vi "Main.vi"(8 "error in (no error)":errorcluster, 11 "Retiga in":refnum<class "Retiga.lvclass">) -> (0 "error out":errorcluster, 3 "component":refnum<class "Retiga.lvclass">)   [LabVIEW 2012, in "Retiga.lvclass"]
doc: "Main VI of the component. This should contain the GUI of your component and be called when creating an executable."
uses:
  Retiga.lvclass
  <vilib>/Distrio/Murmex/Murmex/command_enum.ctl
  <vilib>/Distrio/Murmex/InitialiseMessage/InitialiseMessage.lvclass
  <vilib>/Distrio/Murmex/TerminateMessage/TerminateMessage.lvclass
  <vilib>/Distrio/Murmex/ConfigureMessage/ConfigureMessage.lvclass
  <vilib>/Distrio/Murmex/StopMessage/StopMessage.lvclass
  <vilib>/Distrio/Murmex/StartMessage/StartMessage.lvclass
  <vilib>/Distrio/Murmex/Murmex/update_cluster.ctl
  <vilib>/Distrio/Murmex/GenericMessage/GenericMessage.lvclass
  Retiga.lvclass/Retiga.ctl
  <vilib>/Distrio/Murmex/Murmex/Murmex.lvclass
  <vilib>/Distrio/Murmex/Murmex/Set configure at initialise.vi
  <vilib>/Distrio/Murmex/Murmex/Set log reference.vi
  <vilib>/Distrio/Murmex/Murmex/Set VI reference.vi
  <vilib>/Distrio/Murmex/Murmex/Get ID.vi
  <vilib>/Distrio/Murmex/Murmex/Set write log to disk.vi
  <vilib>/Distrio/Murmex/Message/Add or replace parameter.vi
  <vilib>/Distrio/Murmex/Message/Message.lvclass
panel:
  in  "PID gains":T1
  out "terminate?":bool
  in  "button:configure":bool
  in  "button:quit":bool
  in  "Tab Control":enum32{"Focus", "Phase comparison", "Debug"}(tab)
  in  "button:select_rois":bool
  in  "button:save":bool
  in  "button:start":bool
  in  "File Name":string
  in  "Base Path":path
  in  "Exposure (us)":i32
  in  "Gain":i32
  out "Focus":T2(plugin-control)
  out "av. translation":dbl[unit]
  in  "button:send move":bool
  in  "button:autofocus":bool
  in  "button:set as focus":bool
  out "aligned":T2(plugin-control)
  out "roy":T2(plugin-control)
  out "rob":T2(plugin-control)
  out "ROY":T2(plugin-control)
  out "ROB":T2(plugin-control)
  out "good alignment?":bool
  out "translation":dbl[unit]
  out "pixel shift":dbl
  out "log":string
  in  "Component id":string="Retiga"
  in  "command":T3
  in  "generic command":string
  in  "button:send command":bool
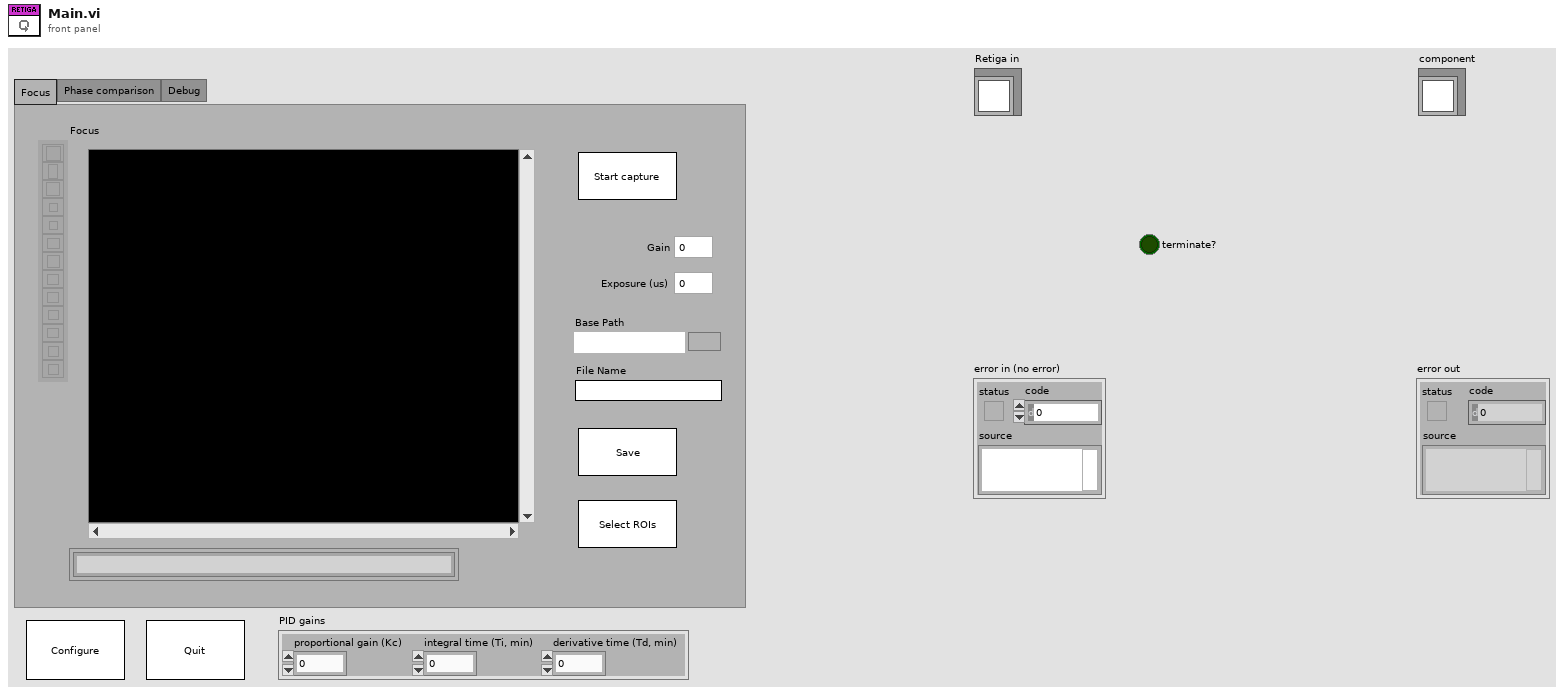
[diagram p1: front panel]
types:
  T1 = cluster{"proportional gain (Kc)":dbl, "integral time (Ti, min)":dbl, "derivative time (Td, min)":dbl}
  T2 = typedef "IMAQ Image.ctl" = refnum<image>
  T3 = typedef "Murmex.lvlib/Murmex.lvclass/command_enum.ctl" = enum16{"null", "initialise", "reset", "terminate", "acknowledge", "update", "inspect", "inform", "proceed", "start", "stop", "fetch", "configure", "generic"}
  T4 = enum8{"Enabled", "Disabled", "Disabled and Grayed Out"}
  T5 = typedef "Murmex.lvlib/Murmex.lvclass/update_cluster.ctl" = cluster{"target ID":string, "key chains":string[], "values":variant[]}
  T6 = typedef "Murmex.lvclass/command_enum.ctl" = enum16{"null", "initialise", "reset", "terminate", "acknowledge", "update", "inspect", "inform", "proceed", "start", "stop", "fetch", "configure", "generic"}
  T7 = typedef "Murmex.lvclass/Event type enumerations.ctl" = enum16{"before", "after"}
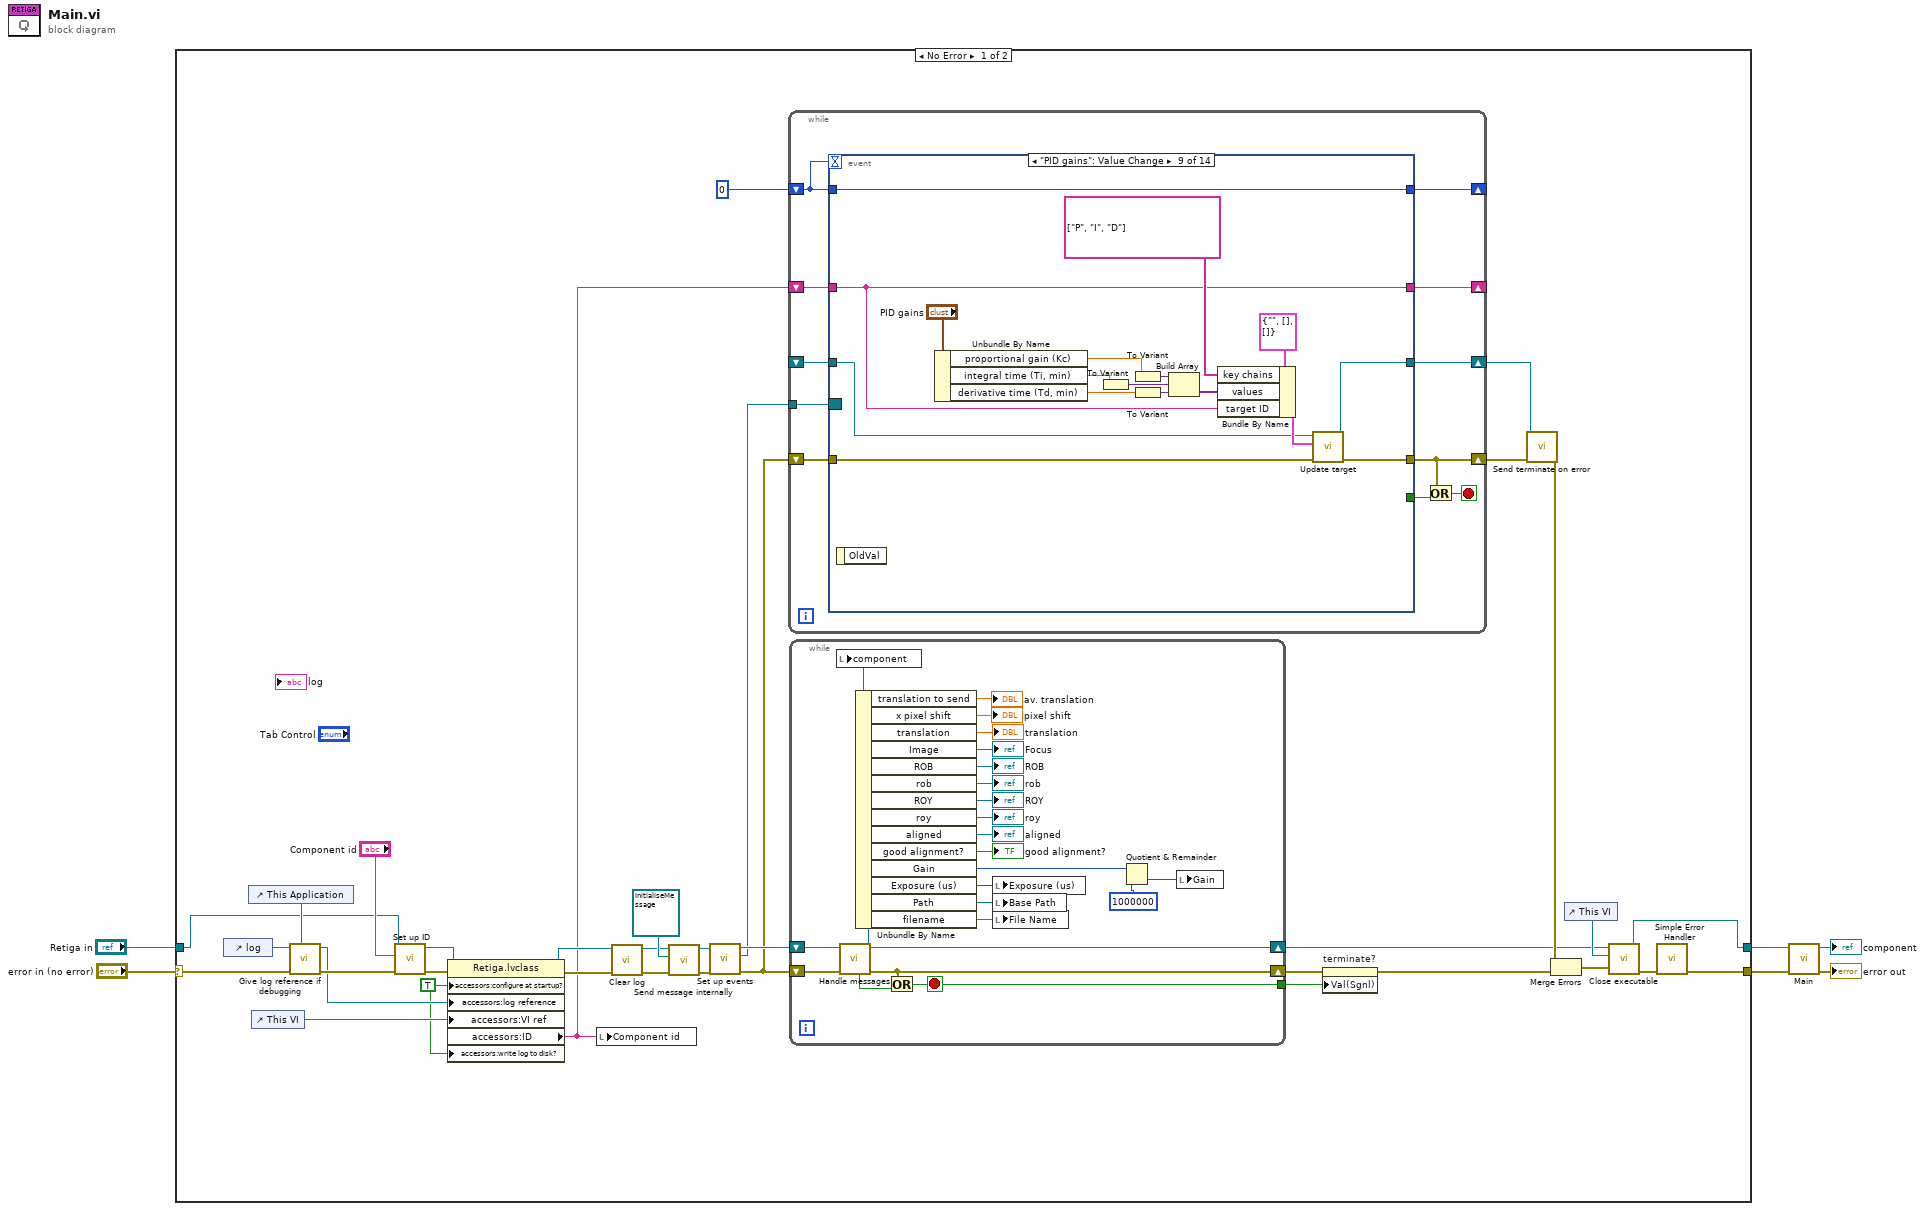
[diagram p0: block diagram]
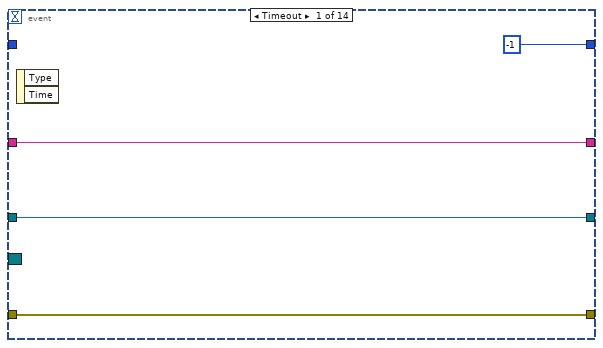
[diagram p2: hidden frame]
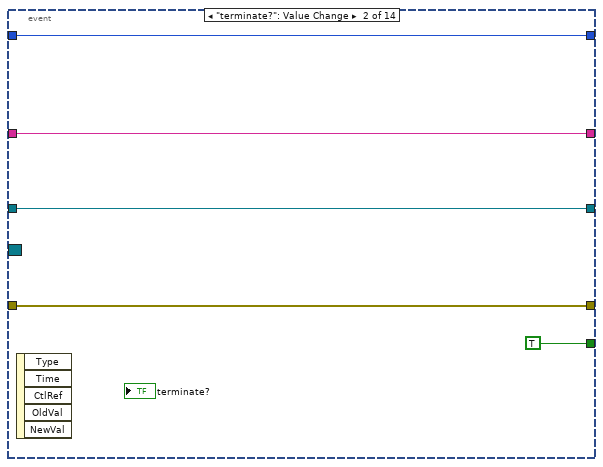
[diagram p3: hidden frame]
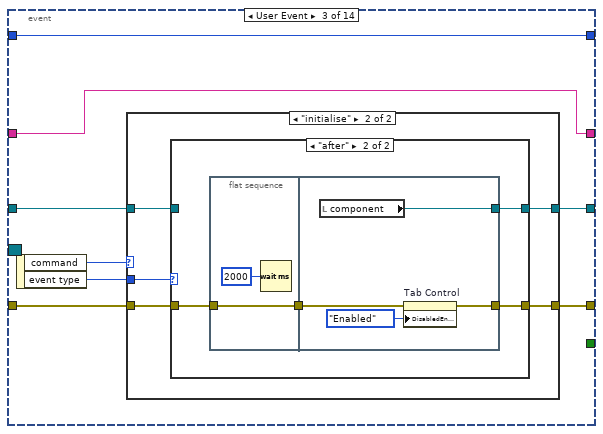
[diagram p4: hidden frame]
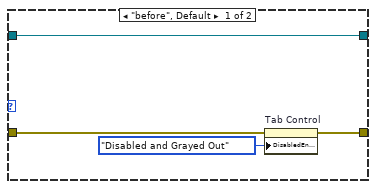
[diagram p6: hidden frame]
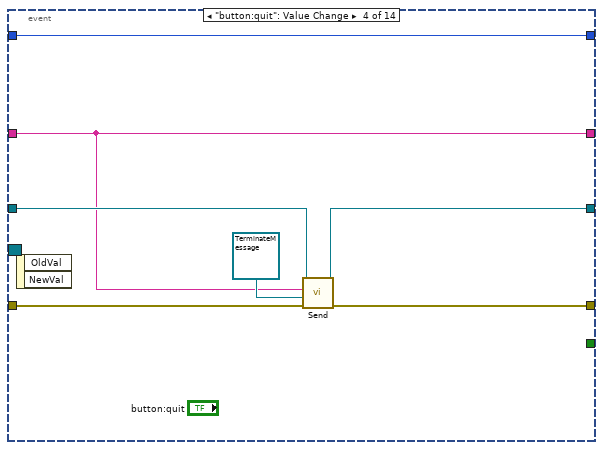
[diagram p7: hidden frame]
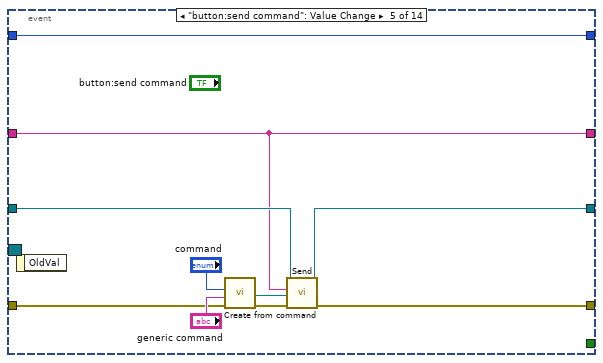
[diagram p8: hidden frame]
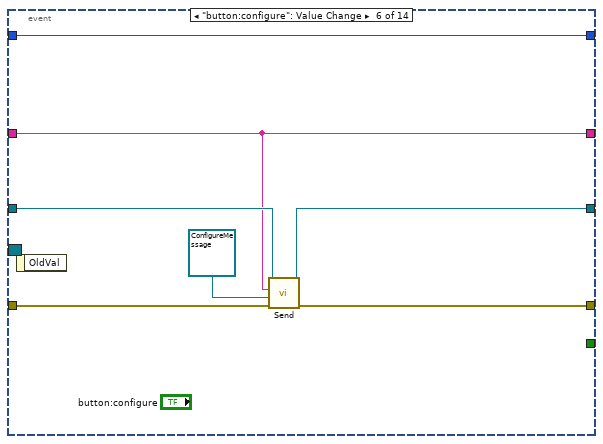
[diagram p9: hidden frame]
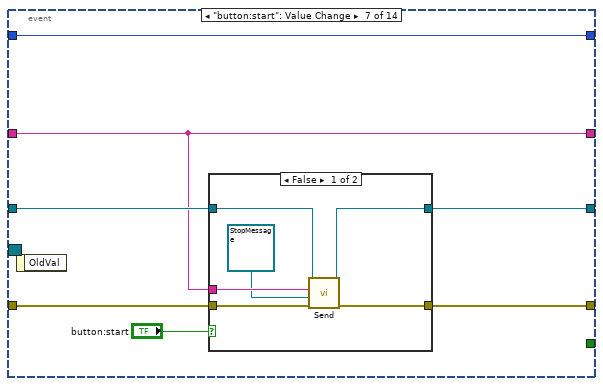
[diagram p10: hidden frame]
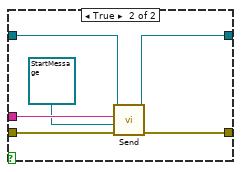
[diagram p11: hidden frame]
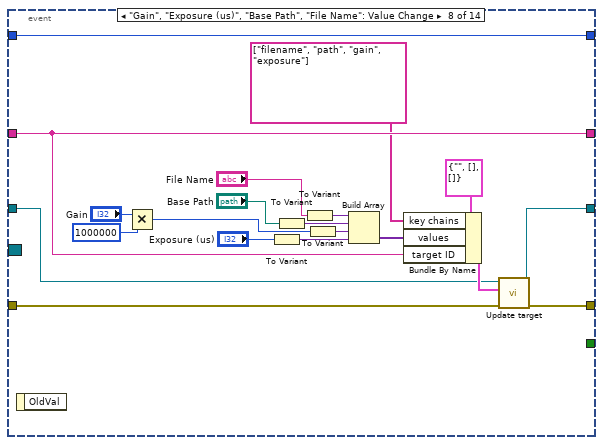
[diagram p12: hidden frame]
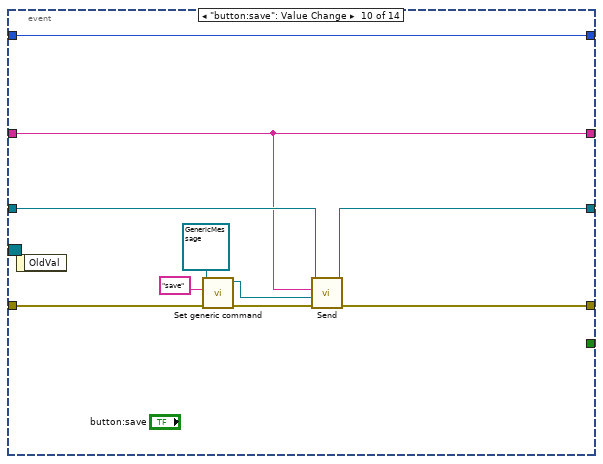
[diagram p13: hidden frame]
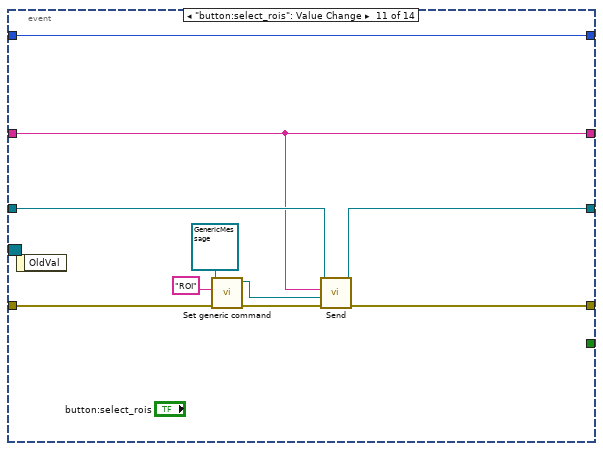
[diagram p14: hidden frame]
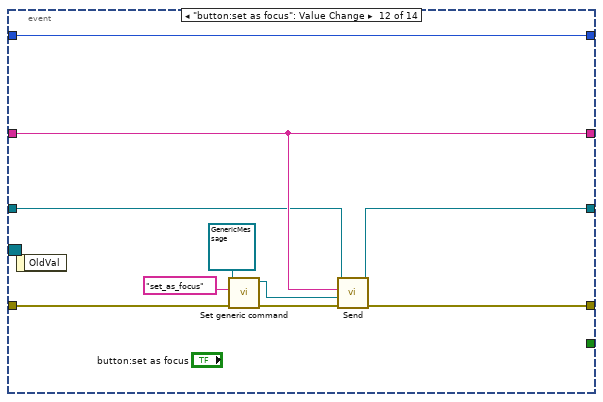
[diagram p15: hidden frame]
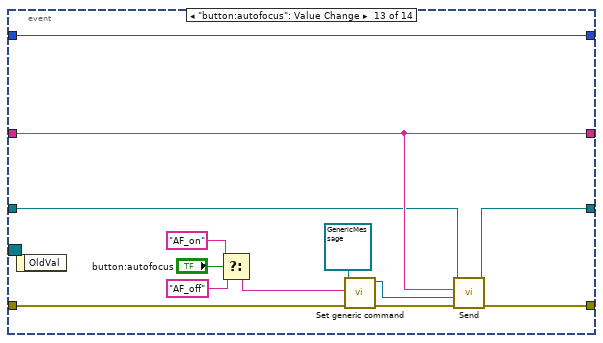
[diagram p16: hidden frame]
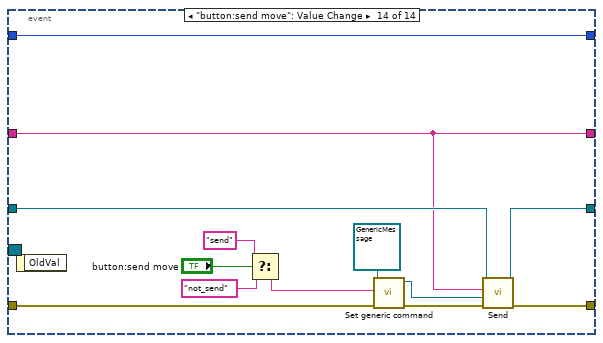
[diagram p17: hidden frame]
diagram:
  n1 = case shown="No Error" "error in (no error)" {
    selector: "error in (no error)" -> [w31 w249]
    tunnel: "Retiga in" -> [w32 w250]
    tunnel: [w13 w250] -> w2
    tunnel: [w14 w249] -> w1
    frame No Error {
      w33 = TRUE ("configure at startup?")
      n2 = control-ref of="log"() -> (w35:refnum<vi>)
      n3 = control-ref of="This Application"() -> (w41:refnum<vi>)
      n4 = control-ref of="This VI"() -> (w34:refnum<vi>)
      n5 = call "Give log reference if debugging.vi"("application ref"=w41, "error in (no error)"=w31, "log reference in"=w35) -> ("error out"=w40:errorcluster, "log reference out"=w36:refnum<vi>)  [unwired: 6 in, 1 out]
      n6 = call <vilib>:"Set up ID.vi"("error in (no error)"=w40, "component ID"="Component id", "MurmexBase in"=w32) -> ("error out"=w38:errorcluster, "MurmexBase out"=w37:refnum<class "Retiga.lvclass">)  [unwired: 6 in, 1 out]
      n7 = property class="Retiga.lvclass"(reference=w37, error in=w38, "accessors:configure at startup?"=w33, "accessors:log reference"=w36, "accessors:VI ref"=w34, "accessors:write log to disk?"=w33) -> (reference out=w24:refnum<class "Retiga.lvclass">, error out=w25:errorcluster, "accessors:ID"=w20:string)
      n8 = local write "Component id"(w20) -> ()
      n9 = call <vilib>:"Clear log.vi"("error in (no error)"=w25, "MurmexBase in"=w24) -> ("error out"=w27:errorcluster, "MurmexBase out"=w26:refnum<class "Retiga.lvclass">)  [unwired: 8 in]
      n10 = call <vilib>:"Send message internally.vi"("error in (no error)"=w27, "Message"=refnum<class "InitialiseMessage.lvclass"> refnum ("InitialiseMessage"), "Murmex in"=w26) -> ("error out"=w28:errorcluster, "Murmex out"=w29:refnum<class "Retiga.lvclass">)  [unwired: 7 in]
      n11 = call <vilib>:"Set up events.vi"("error in (no error)"=w28, "MurmexBase in"=w29) -> ("error out"=w21:errorcluster, "Event Registration Refnum"=w19:refnum<event-registration>, "MurmexBase out"=w23:refnum<class "Retiga.lvclass">)  [unwired: 7 in]
      n12 = while {
        shift-right: [w51] -> _
        shift-left: 0 -> [w52]
        shift-right: [w46] -> w11
        shift-left: w21 -> [w50]
        shift-right: [w48] -> _
        shift-left: w20 -> [w49]
        tunnel: w19 -> [w47]
        shift-right: [w43] -> w10
        shift-left: _ -> [w42]
        stop <- w44 stop-if-true
        n13 = event shown="[8] \"PID gains\": Value Change" {
          selector: w47 -> [_ _ _ _ _ _ _ _ _ _ _ _ _ _]
          dyn-events: _ -> [_ _ _ _ _ _ _ _ _ _ _ _ _ _]
          timeout: w52 -> [_ _ _ _ _ _ _ _ _ _ _ _ _ _]
          tunnel: w52 -> [_ w58 w62 w91 w99 w108 w115 w145 w158 w171 w181 w195 w201 w215]
          tunnel: [-1 w58 w62 w91 w99 w108 w115 w145 w158 w171 w181 w195 w201 w215] -> w51
          tunnel: w50 -> [w55 w60 w66 w97 w103 w113 w119 w149 w163 w177 w187 w198 w210 w220]
          tunnel: [w55 w60 w65 w96 w102 w112 w118 w148 w162 w175 w185 w196 w209 w219] -> w46
          tunnel: w49 -> [w54 w59 w63 w92 w98 w109 w116 w146 w159 w172 w182 w194 w207 w216]
          tunnel: [w54 w59 w63 w92 w98 w109 w116 w146 w159 w172 w182 w194 w207 w216] -> w48
          tunnel: [_ TRUE _ _ _ _ _ _ _ _ _ _ _ _] -> w45
          tunnel: [w53 w57 w67 w93 w100 w110 w120 w144 w160 w173 w183 w192 w208 w218] -> w43
          tunnel: w42 -> [w53 w57 w64 w94 w101 w111 w121 w147 w161 w174 w184 w193 w206 w217]
          event Timeout {
            n14 = event-data() -> ()  [unwired: 1 in, 2 out]
          }
          event "terminate?": Value Change {
            n15 = event-data() -> ()  [unwired: 1 in, 5 out]
          }
          event User Event {
            n16 = event-data() -> ("command"=w69:T6, "event type"=w68:T7)  [unwired: 1 in]
            n17 = case shown="\"initialise\"" w69 {
              tunnel: w68 -> [_ w76]
              tunnel: [w71 w75] -> w67
              tunnel: w66 -> [w70 w74]
              tunnel: [w70 w73] -> w65
              tunnel: w64 -> [w71 w72]
              frame "null", Default {
              }
              frame "initialise" {
                n18 = case shown="\"after\"" w76 {
                  tunnel: [w80 w84] -> w75
                  tunnel: w74 -> [w79 w82]
                  tunnel: [w78 w81] -> w73
                  tunnel: w72 -> [w80 _]
                  frame "before", Default {
                    n19 = property on="Tab Control" class="TabCtl (strict)"(error in=w79, "DisabledEnum"=T4."Disabled and Grayed Out" ("Disabled")) -> (error out=w78:errorcluster)  [unwired: 1 in, 1 out]
                  }
                  frame "after" {
                    n20 = flat-sequence {
                      tunnel: [w85] -> w83
                      tunnel: w82 -> [w85]
                      tunnel: [w90] -> w84
                      tunnel: w83 -> [w89]
                      tunnel: [w87] -> w81
                      frame #0 {
                        n21 = Wait (ms)(milliseconds to wait=u32 2000) -> ()  [unwired: 1 out]
                      }
                      frame #1 {
                        n22 = local read "component"() -> (w90:refnum<class "Retiga.lvclass">)
                        n23 = property on="Tab Control" class="TabCtl (strict)"(error in=w89, "DisabledEnum"=T4."Enabled" ("Disabled")) -> (error out=w87:errorcluster)  [unwired: 1 in, 1 out]
                      }
                    }
                  }
                }
              }
            }
          }
          event "button:quit": Value Change {
            n24 = event-data() -> ()  [unwired: 1 in, 2 out]
            n25 = call <vilib>:"Send.vi"("error in (no error)"=w97, "Message"=refnum<class "TerminateMessage.lvclass"> refnum ("TerminateMessage"), "recipient"=w92, "Murmex in"=w94) -> ("error out"=w96:errorcluster, "Murmex out"=w93:refnum<class "Retiga.lvclass">)  [unwired: 6 in]
          }
          event "button:send command": Value Change {
            n26 = event-data() -> ()  [unwired: 1 in, 1 out]
            n27 = call <vilib>:"Create from command.vi"("error in (no error)"=w103, "generic command"="generic command", "command"="command") -> ("error out"=w107:errorcluster, "Message out"=w104:refnum<class "Message.lvclass">)  [unwired: 7 in]
            n28 = call <vilib>:"Send.vi"("error in (no error)"=w107, "Message"=w104, "recipient"=w98, "Murmex in"=w101) -> ("error out"=w102:errorcluster, "Murmex out"=w100:refnum<class "Retiga.lvclass">)  [unwired: 6 in]
          }
          event "button:configure": Value Change {
            n29 = event-data() -> ()  [unwired: 1 in, 1 out]
            n30 = call <vilib>:"Send.vi"("error in (no error)"=w113, "Message"=refnum<class "ConfigureMessage.lvclass"> refnum ("ConfigureMessage"), "recipient"=w109, "Murmex in"=w111) -> ("error out"=w112:errorcluster, "Murmex out"=w110:refnum<class "Retiga.lvclass">)  [unwired: 6 in]
          }
          event "button:start": Value Change {
            n31 = event-data() -> ()  [unwired: 1 in, 1 out]
            n32 = case shown="False" "button:start" {
              tunnel: w116 -> [w126 w133]
              tunnel: w121 -> [w123 w132]
              tunnel: [w124 w131] -> w120
              tunnel: w119 -> [w127 w130]
              tunnel: [w125 w129] -> w118
              frame False {
                n33 = call <vilib>:"Send.vi"("error in (no error)"=w127, "Message"=refnum<class "StopMessage.lvclass"> refnum ("Distrio Murmex 1.5:StopMessage"), "recipient"=w126, "Murmex in"=w123) -> ("error out"=w125:errorcluster, "Murmex out"=w124:refnum<class "Retiga.lvclass">)  [unwired: 6 in]
              }
              frame True {
                n34 = call <vilib>:"Send.vi"("error in (no error)"=w130, "Message"=refnum<class "StartMessage.lvclass"> refnum ("Distrio Murmex 1.5:StartMessage"), "recipient"=w133, "Murmex in"=w132) -> ("error out"=w129:errorcluster, "Murmex out"=w131:refnum<class "Retiga.lvclass">)  [unwired: 6 in]
              }
            }
          }
          event "Gain", "Exposure (us)", "Base Path", "File Name": Value Change {
            n35 = event-data() -> ()  [unwired: 1 in, 1 out]
            n36 = Multiply(x="Gain", y=1000000) -> (x*y=w135:i32)
            n37 = To Variant(anything="Exposure (us)") -> (Variant=w152:variant)
            n38 = To Variant(anything="Base Path") -> (Variant=w141:variant)
            n39 = To Variant(anything="File Name") -> (Variant=w143:variant)
            n40 = To Variant(anything=w135) -> (Variant=w142:variant)
            n41 = Build Array(w143, w141, w142, w152) -> (w153:variant[])
            n42 = Bundle By Name(cluster=T5 {"target ID"="", "key chains"=[], "values"=[]} ("update cluster"), "key chains"=string[] ["filename", "path", "gain", "exposure"], "values"=w153, "target ID"=w146) -> (w150:T5)
            n43 = call <vilib>:"Update target.vi"("error in (no error)"=w149, "update cluster"=w150, "MurmexBase in"=w147) -> ("error out"=w148:errorcluster, "MurmexBase out"=w144:refnum<class "Retiga.lvclass">)  [unwired: 7 in]
          }
          event "PID gains": Value Change {
            n44 = event-data() -> ()  [unwired: 1 in, 1 out]
            n45 = Unbundle By Name("PID gains") -> ("proportional gain (Kc)"=w156:dbl, "integral time (Ti, min)"=w155:dbl, "derivative time (Td, min)"=w154:dbl)
            n46 = To Variant(anything=w155) -> (Variant=w165:variant)
            n47 = To Variant(anything=w156) -> (Variant=w167:variant)
            n48 = To Variant(anything=w154) -> (Variant=w166:variant)
            n49 = Build Array(w167, w165, w166) -> (w170:variant[])
            n50 = Bundle By Name(cluster=T5 {"target ID"="", "key chains"=[], "values"=[]} ("update cluster"), "key chains"=string[] ["P", "I", "D"], "values"=w170, "target ID"=w159) -> (w168:T5)
            n51 = call <vilib>:"Update target.vi"("error in (no error)"=w163, "update cluster"=w168, "MurmexBase in"=w161) -> ("error out"=w162:errorcluster, "MurmexBase out"=w160:refnum<class "Retiga.lvclass">)  [unwired: 7 in]
          }
          event "button:save": Value Change {
            n52 = event-data() -> ()  [unwired: 1 in, 1 out]
            n53 = call <vilib>:"Set generic command.vi"("error in (no error)"=w177, "generic command"="save", "GenericMessage in"=refnum<class "GenericMessage.lvclass"> refnum ("Message in")) -> ("error out"=w176:errorcluster, "GenericMessage out"=w179:refnum<class "GenericMessage.lvclass">)  [unwired: 7 in]
            n54 = call <vilib>:"Send.vi"("error in (no error)"=w176, "Message"=w179, "recipient"=w172, "Murmex in"=w174) -> ("error out"=w175:errorcluster, "Murmex out"=w173:refnum<class "Retiga.lvclass">)  [unwired: 6 in]
          }
          event "button:select_rois": Value Change {
            n55 = event-data() -> ()  [unwired: 1 in, 1 out]
            n56 = call <vilib>:"Set generic command.vi"("error in (no error)"=w187, "generic command"="ROI", "GenericMessage in"=refnum<class "GenericMessage.lvclass"> refnum ("Message in")) -> ("error out"=w186:errorcluster, "GenericMessage out"=w189:refnum<class "GenericMessage.lvclass">)  [unwired: 7 in]
            n57 = call <vilib>:"Send.vi"("error in (no error)"=w186, "Message"=w189, "recipient"=w182, "Murmex in"=w184) -> ("error out"=w185:errorcluster, "Murmex out"=w183:refnum<class "Retiga.lvclass">)  [unwired: 6 in]
          }
          event "button:set as focus": Value Change {
            n58 = event-data() -> ()  [unwired: 1 in, 1 out]
            n59 = call <vilib>:"Set generic command.vi"("error in (no error)"=w198, "generic command"="set_as_focus", "GenericMessage in"=refnum<class "GenericMessage.lvclass"> refnum ("Message in")) -> ("error out"=w197:errorcluster, "GenericMessage out"=w191:refnum<class "GenericMessage.lvclass">)  [unwired: 7 in]
            n60 = call <vilib>:"Send.vi"("error in (no error)"=w197, "Message"=w191, "recipient"=w194, "Murmex in"=w193) -> ("error out"=w196:errorcluster, "Murmex out"=w192:refnum<class "Retiga.lvclass">)  [unwired: 6 in]
          }
          event "button:autofocus": Value Change {
            n61 = event-data() -> ()  [unwired: 1 in, 1 out]
            n62 = Select(t="AF_on" ("generic command"), s="button:autofocus", f="AF_off" ("generic command")) -> (s? t:f=w202:string)
            n63 = call <vilib>:"Set generic command.vi"("error in (no error)"=w210, "generic command"=w202, "GenericMessage in"=refnum<class "GenericMessage.lvclass"> refnum ("Message in")) -> ("error out"=w212:errorcluster, "GenericMessage out"=w211:refnum<class "GenericMessage.lvclass">)  [unwired: 7 in]
            n64 = call <vilib>:"Send.vi"("error in (no error)"=w212, "Message"=w211, "recipient"=w207, "Murmex in"=w206) -> ("error out"=w209:errorcluster, "Murmex out"=w208:refnum<class "Retiga.lvclass">)  [unwired: 6 in]
          }
          event "button:send move": Value Change {
            n65 = event-data() -> ()  [unwired: 1 in, 1 out]
            n66 = Select(t="send" ("generic command"), s="button:send move", f="not_send" ("generic command")) -> (s? t:f=w221:string)
            n67 = call <vilib>:"Set generic command.vi"("error in (no error)"=w220, "generic command"=w221, "GenericMessage in"=refnum<class "GenericMessage.lvclass"> refnum ("Message in")) -> ("error out"=w225:errorcluster, "GenericMessage out"=w224:refnum<class "GenericMessage.lvclass">)  [unwired: 7 in]
            n68 = call <vilib>:"Send.vi"("error in (no error)"=w225, "Message"=w224, "recipient"=w216, "Murmex in"=w217) -> ("error out"=w219:errorcluster, "Murmex out"=w218:refnum<class "Retiga.lvclass">)  [unwired: 6 in]
          }
        }
        n69 = Or(x=w46, y=w45) -> (x .or. y?=w44:bool)
      }
      n70 = while {
        shift-right: [w245] -> w9
        shift-left: w21 -> [w247]
        shift-right: [w243] -> w12
        shift-left: w23 -> [w248]
        tunnel: [w244] -> w7
        stop <- w244 stop-if-true
        n71 = call <vilib>:"Handle messages.vi"("error in (no error)"=w247, "Murmex in"=w248) -> ("error out"=w245:errorcluster, "Murmex out"=w243:refnum<class "Retiga.lvclass">, "terminated?"=w246:bool)  [unwired: 7 in]
        n72 = local write "component"(w243) -> ()
        n73 = Unbundle By Name(w243) -> ("translation to send"=→"av. translation":dbl[unit], "x pixel shift"=→"pixel shift":dbl, "translation"=→"translation":dbl[unit], "Image"=→"Focus":T2, "ROB"=→"ROB":T2, "rob"=→"rob":T2, "ROY"=→"ROY":T2, "roy"=→"roy":T2, "aligned"=→"aligned":T2, "good alignment?"=→"good alignment?":bool, "Gain"=w229:i32, "Exposure (us)"=w241:i32, "Path"=w233:path, "filename"=w242:string)
        n74 = Or(x=w245, y=w246) -> (x .or. y?=w244:bool)
        n75 = local write "Exposure (us)"(w241) -> ()
        n76 = local write "Base Path"(w233) -> ()
        n77 = local write "File Name"(w242) -> ()
        n78 = Quotient & Remainder(x=w229, y=1000000) -> (floor(x/y)=w228:i32)  [unwired: 1 out]
        n79 = local write "Gain"(w228) -> ()
      }
      n80 = property on="terminate?" class="Bool (strict)"(error in=w9, "Val(Sgnl)"=w7) -> (error out=w8:errorcluster)  [unwired: 1 in, 1 out]
      n81 = call <vilib>:"Send terminate on error.vi"("error in (no error)"=w11, "Murmex in"=w10) -> ("error out"=w15:errorcluster)  [unwired: 8 in, 1 out]
      n82 = Merge Errors(w15, w8) -> (w17:errorcluster)
      n83 = control-ref of="This VI"() -> (w16:refnum<vi>)
      n84 = call <vilib>:"Close executable.vi"("error in (no error)"=w17, "main VI ref (optional)"=w16, "MurmexBase in"=w12) -> ("error out"=w18:errorcluster, "MurmexBase out"=w13:refnum<class "Retiga.lvclass">)  [unwired: 7 in]
      n85 = call <vilib>:"Simple Error Handler.vi"("error in (no error)"=w18) -> ("error out"=w14:errorcluster)  [unwired: 4 in, 4 out]
    }
    frame Error {
    }
  }
  n86 = call-parent "Main.vi"("error in (no error)"=w1, "Murmex in"=w2) -> ("error out"=→"error out":errorcluster, "Murmex out"=→"component":refnum<class "Retiga.lvclass">)  [unwired: 8 in]
